vi "laseranswer.vi"(1 "IN":string) -> (0 "Answer":string)   [LabVIEW 2011]
uses:
  <vilib>/regexp/Match Regular Expression.xnode
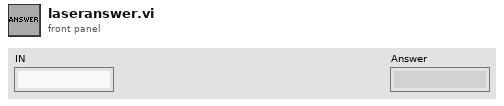
[diagram p1: front panel]
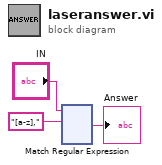
[diagram p0: block diagram]
diagram:
  n1 = xnode "Match Regular Expression"("input string"="IN", "regular expression"="[a-z],") -> ("after match"=→"Answer":string)  [unwired: 4 in, 4 out]
